vi "model selection.vi"(11 "file path (use dialog)":path=path "D:/data/Test Settings") -> (2 "OK":bool, 3 "Test Name 2":string)   [LabVIEW 2024]
panel:
  in  "OK 2":bool
  in  "Cancel":bool
  out "Date and Time:":string="10/20/2014   5:08:59 PM"
  in  "Model  Name":string(combo)
  # "Please Select Model Name"
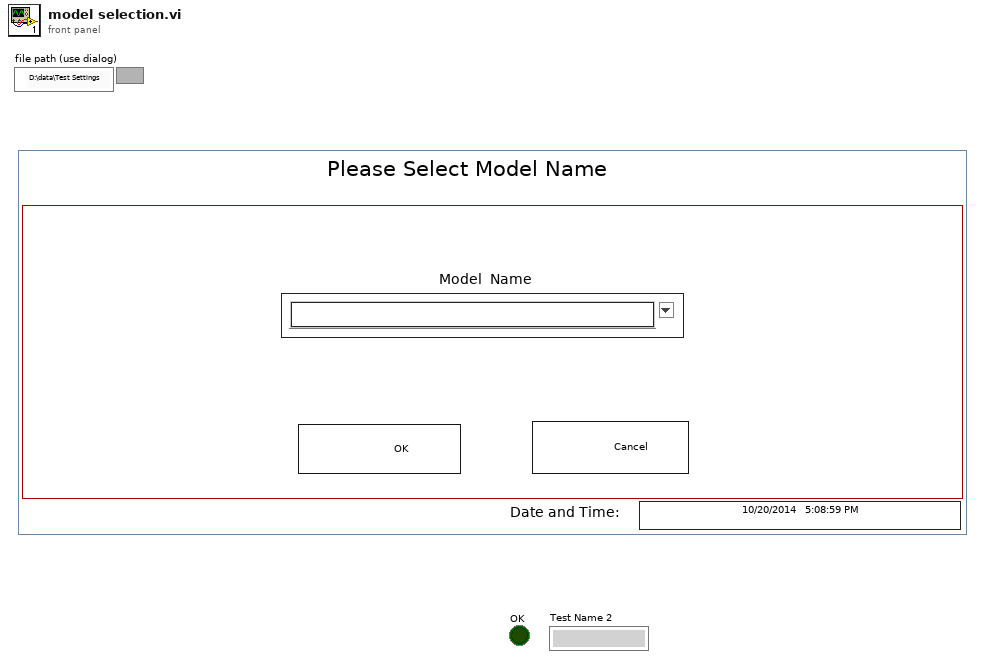
[diagram p1: front panel]
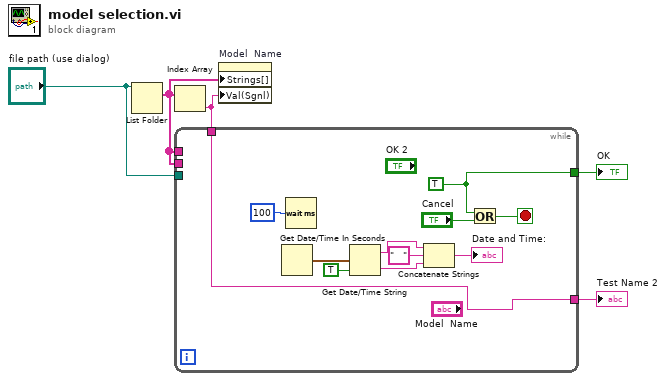
[diagram p0: block diagram]
diagram:
  n1 = List Folder(path="file path (use dialog)") -> (filenames=w3:string[])  [unwired: 3 in, 3 out]
  n2 = Index Array(array=w3) -> (element=w1:string)  [unwired: 1 in]
  n3 = while {
    tunnel: [w7] -> w2
    tunnel: [w6] -> w5
    tunnel: w3 -> [_]
    tunnel: "file path (use dialog)" -> [_]
    tunnel: w3 -> [_]
    tunnel: w1 -> [w6]
    stop <- w16 stop-if-true
    w7 = TRUE ("OK 2")
    n4 = Get Date/Time In Seconds() -> (seconds since 1Jan1904=w12:timestamp)
    n5 = Wait (ms)(milliseconds to wait=u32 100) -> ()  [unwired: 1 out]
    n6 = Get Date/Time String(seconds (now)=w12, want seconds? (F)=TRUE) -> (date string=w9:string, time string=w11:string)  [unwired: 1 in]
    n7 = Concatenate Strings(w9, "   " ("string"), w11) -> (→"Date and Time:":string)
    n8 = Or(x=w7, y="Cancel") -> (x .or. y?=w16:bool)
  }
  "OK" <- w2
  "Test Name 2" <- w5
  n9 = property on="Model  Name" class="CmbBox"("Strings[]"=w3, "Val(Sgnl)"=w1) -> ()  [unwired: 2 in, 2 out]
